vi "intensity_show_image.vi"() -> ()   [LabVIEW 2022 SP3]
panel:
  out "Intensity Graph B":u8[][](graph)
  out "Intensity Graph G":u8[][](graph)
  out "Intensity Graph R":u8[][](graph)
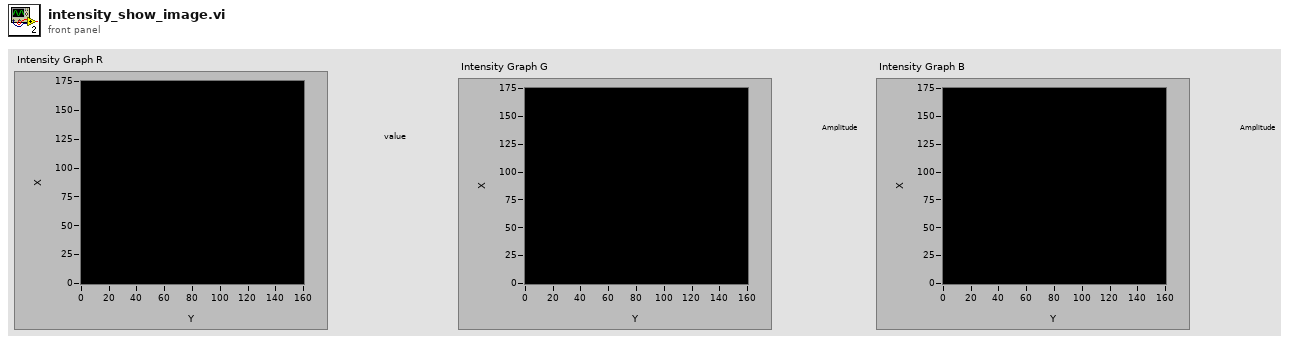
[diagram p1: front panel]
types:
  T1 = typedef "imagedata.ctl" = cluster{"image type":i32, "image depth":i32, "image":u8[], "mask":u8[], "colors":u32[], "Rectangle":cluster{"left":i16, "top":i16, "right":i16, "bottom":i16}}
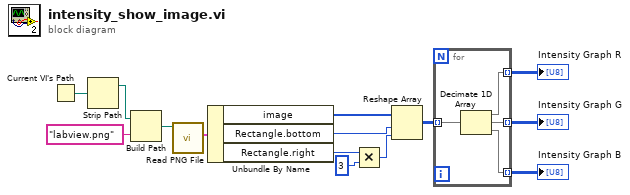
[diagram p0: block diagram]
diagram:
  n1 = Current VI's Path() -> (path=w12:path)
  n2 = Strip Path(path=w12) -> (stripped path=w13:path)  [unwired: 1 out]
  n3 = Build Path(base path=w13, name or relative path="labview.png") -> (appended path=w11:path)
  n4 = call <vilib>:"Read PNG File.vi"("path to PNG file"=w11) -> ("image data"=w10:T1)  [unwired: 8 in, 2 out]
  n5 = Unbundle By Name(w10) -> ("image"=w9:u8[], "Rectangle.bottom"=w7:i16, "Rectangle.right"=w6:i16)
  n6 = Multiply(x=w6, y=i16 3) -> (x*y=w5:i16)
  n7 = Reshape Array(w9, w7, w5) -> (w4:u8[][])
  n8 = for {
    tunnel: w4 -> [w18] mode=indexing
    tunnel: [w17] -> w3 mode=indexing
    tunnel: [w16] -> w2 mode=indexing
    tunnel: [w15] -> w1 mode=indexing
    n9 = Decimate 1D Array(w18) -> (w17:u8[], w16:u8[], w15:u8[])
  }
  "Intensity Graph R" <- w3
  "Intensity Graph G" <- w2
  "Intensity Graph B" <- w1
